vi "displayXMLExpresssion.vi"(10 "xmlParser 0":string[](array[string]), 11 "String in":string) -> (3 "String out":string)   [LabVIEW 2018]
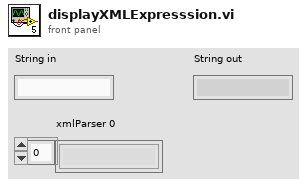
[diagram p1: front panel]
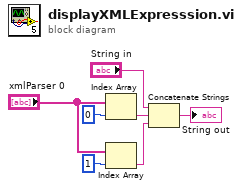
[diagram p0: block diagram]
diagram:
  n1 = Index Array(array="xmlParser 0", index=0) -> (element=w2:string)
  n2 = Index Array(array="xmlParser 0", index=1) -> (element=w6:string)
  n3 = Concatenate Strings("String in", w2, w6) -> (→"String out":string)
